vi "Execute.vi"(7 "{{Name}}Message":refnum<class "{{Name}}Message.lvclass">, 8 "Error":errorcluster, 11 "Actor":refnum<class "Actor.lvclass">) -> (0 "Error":errorcluster, 3 "Actor":refnum<class "Actor.lvclass">, 5 "{{Name}}Message":refnum<class "{{Name}}Message.lvclass">)   [LabVIEW 2020, in "_Template.lvlib" / "Templates.lvlib" / "{{Name}}Message.lvlib" / "{{Name}}Message.lvclass"]
uses:
  {{Name}}Message.lvclass
  {{Name}}Message.lvclass/{{Name}}Message.ctl
  {{Name}}/{{Name}}.lvclass
  jettl/jettl/Actor/Actor.lvclass
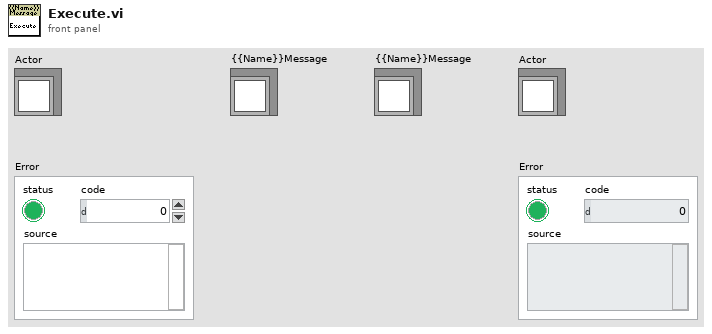
[diagram p1: front panel]
types:
  T1 = typedef "_Template.lvlib/Templates.lvlib/{{Name}}Message.lvlib/Message.ctl" = cluster{"MessageMetadata":T2}
  T2 = typedef "jettl.lvlib/MessageMetadata.ctl" = cluster{"ActorAlias":string, "ActorRelation":T3, "ActorLifetime":T4, "AbsoluteTime":timestamp, "RelativeTime":dbl}
  T3 = typedef "jettl.lvlib/ActorRelation.ctl" = enum16{"Self", "Actor"}
  T4 = typedef "jettl.lvlib/ActorLifetime.ctl" = enum16{"Init", "Spawn", "Setup", "Teardown Before Running", "Running", "Stop Called", "Stopping With Children", "Stopping Without Children", "Teardown After Running", "Stopped"}
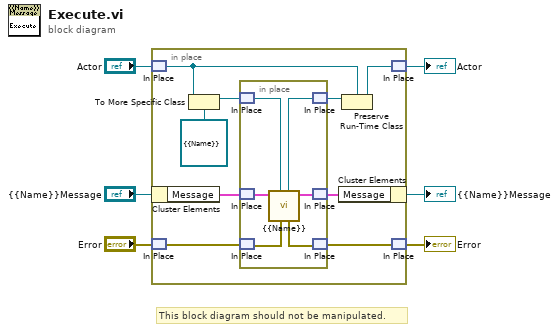
[diagram p0: block diagram]
diagram:
  # "This block diagram should not be manipulated."
  n1 = in-place {
    n2 = in-place-match #1("Actor") -> (w11:refnum<class "Actor.lvclass">)
    n3 = in-place-cluster #2("{{Name}}Message") -> ("Message"=w8:T1)
    n4 = in-place-match #3("Error") -> (w15:errorcluster)
    n5 = To More Specific Class(target class=refnum<class "{{Name}}.lvclass"> refnum ("_Template.lvlib:Templates.lvlib:TEMPLATE jettl Msg.lvlib:TEMPLATE jettl Msg.lvclass"), reference=w11) -> (specific class reference=w12:refnum<class "{{Name}}.lvclass">)  [unwired: 1 in, 1 out]
    n6 = in-place {
      n7 = in-place-match #4(w12) -> (w19:refnum<class "{{Name}}.lvclass">)
      n8 = in-place-match #5(w8) -> (w17:T1)
      n9 = in-place-match #6(w15) -> (w21:errorcluster)
      n10 = call-dynamic "{{Name}}.vi"("Error in"=w21, 7:"{{Name}}"=w19, 11:"{{Name}}"=w17) -> (3:"{{Name}}"=w16:T1, "Error out"=w20:errorcluster, 5:"{{Name}}"=w18:refnum<class "{{Name}}.lvclass">)  [unwired: 6 in]
      n11 = in-place-match #4(w18) -> (w9:refnum<class "{{Name}}.lvclass">)
      n12 = in-place-match #5(w16) -> (w7:T1)
      n13 = in-place-match #6(w20) -> (w14:errorcluster)
    }
    n14 = in-place-cluster #2("Message"=w7) -> (→"{{Name}}Message":refnum<class "{{Name}}Message.lvclass">)
    n15 = Preserve Run-Time Class(object in=w9, 2:w11) -> (object out=w10:refnum<class "Actor.lvclass">)  [unwired: 1 in, 1 out]
    n16 = in-place-match #1(w10) -> (→"Actor":refnum<class "Actor.lvclass">)
    n17 = in-place-match #3(w14) -> (→"Error":errorcluster)
  }
